vi "Is Inline.vi"(11 "Timing in":refnum<class "Timing.lvclass">) -> (2 "inline?":bool, 3 "Timing out":refnum<class "Timing.lvclass">)   [LabVIEW 2017, in "DSF Core.lvlib" / "Timing.lvclass"]
uses:
  Timing.lvclass
  Timing.lvclass/Timing.ctl
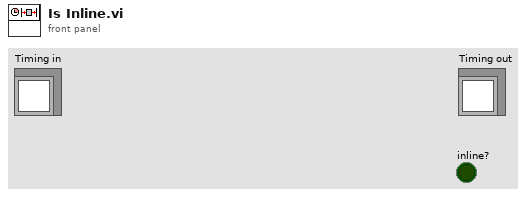
[diagram p1: front panel]
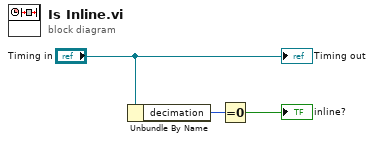
[diagram p0: block diagram]
diagram:
  n1 = Unbundle By Name("Timing in") -> ("decimation"=w2:u64)
  n2 = Equal To 0?(x=w2) -> (x = 0?=→"inline?":bool)
  "Timing out" <- "Timing in"
